vi "Apply Calibration - Slope and Offset.vi"(9 "intercept":dbl, 10 "slope":dbl, 11 "Waveform in":waveform(dbl)) -> (3 "Waveform out":waveform(dbl))   [LabVIEW 2020]
doc: "Scales the strain gauge data by the calibration sensitivity (lbs force/strain gauge volts) and add the calibration offset (lbs)."
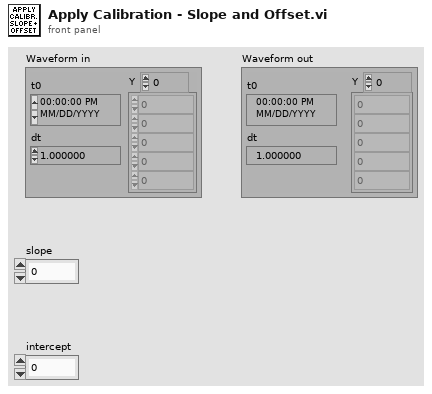
[diagram p1: front panel]
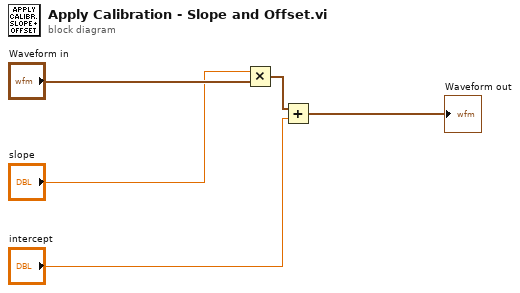
[diagram p0: block diagram]
diagram:
  n1 = Multiply(x="slope", y="Waveform in") -> (x*y=w2:waveform(dbl))
  n2 = Add(x=w2, y="intercept") -> (x+y=→"Waveform out":waveform(dbl))
